vi "Laser_Setup_v1_v19 - Copy.vi"() -> ()   [LabVIEW 2019]
uses:
  <vilib>/Instr/_visa.llb/VISA Configure Serial Port (Instr).vi
panel:
  in  "Message":string
  in  "Arduino Functons":enum32{"DAC", "Step Motors", "TEC", "Settings"}(tab)=enum."Settings"
  in  "DAC: Show outputs value.":bool
  in  "DAC: Set VA.":bool
  in  "DAC: Set VB.":bool
  in  "DAC: Set VC.":bool
  in  "DAC: Set default outputs.":bool
  in  "DAC: Save outputs to DAC.":bool
  in  "DAC: Set VD.":bool
  in  "Step Motors: Reset Motor Y Position.":bool
  in  "Step Motors: Move Motor Y Forward.":bool
  in  "Step Motors: Move Motor X Forward.":bool
  in  "Step Motors: Reset Motor X Position.":bool
  in  "Step Motors: Move Motor Y Backward.":bool
  in  "Step Motors: Move Motor X Backward.":bool
  in  "Step Motors: Show Motor X Position.":bool
  in  "Step Motors: Show Motor Y Position.":bool
  in  "TEC: Get Firmware ID.":bool
  in  "TEC: Get Output Stage Status.":bool
  in  "TEC: Get Device Status.":bool
  in  "TEC: Set Output Stage Status ON.":bool
  in  "TEC: Set Output Stage Status OFF.":bool
  in  "TEC: Get if Temperature is Stable.":bool
  in  "TEC: Get Object Temperature Status.":bool
  in  "TEC: Do a Self Check.":bool
  in  "TEC: Get Error Status.":bool
  in  "TEC: Do Reset.":bool
  in  "TCP Settings":cluster{"Address":string, "Remote port":u16}={"Address"="192.168.4.1", "Remote port"=80}
  in  "Serial Settings":T1={"VISA resource name"="COM1", "baud rate"=9600, "data bits"=8, "parity"=enum."None", "stop bits"=10, "flow control"=0} {"flow control" items=["None"=0, "XON/XOFF"=1, "RTS/CTS"=2, "DTR/DSR"=4]; "stop bits" items=["1.0"=10, "1.5"=15, "2.0"=20]; "data bits" min=5 max=8 step=1; "baud rate" items=["75"=75, "110"=110, "134"=134, "150"=150, "300"=300, "600"=600, "1200"=1200, "1800"=1800, "2400"=2400, "4800"=4800, "7200"=7200, "9600"=9600, "14400"=14400, "19200"=19200, "28800"=28800, "38400"=38400, "56000"=56000, "57600"=57600, "115200"=115200, "128000"=128000, "230400"=230400]}
  in  "Start/Stop Communication":bool
  in  "Default Settings":bool
  in  "Stop VI":bool
  in  "Choose Communication":bool=TRUE
  in  "Main: Start Checks":bool
  out "Response":string
  # "Control Software of Laser Beam Test Bench \nversion 1.0"
  # "National and Kapodistrian University of Athens\nAerospace Inst Lab\n2021"
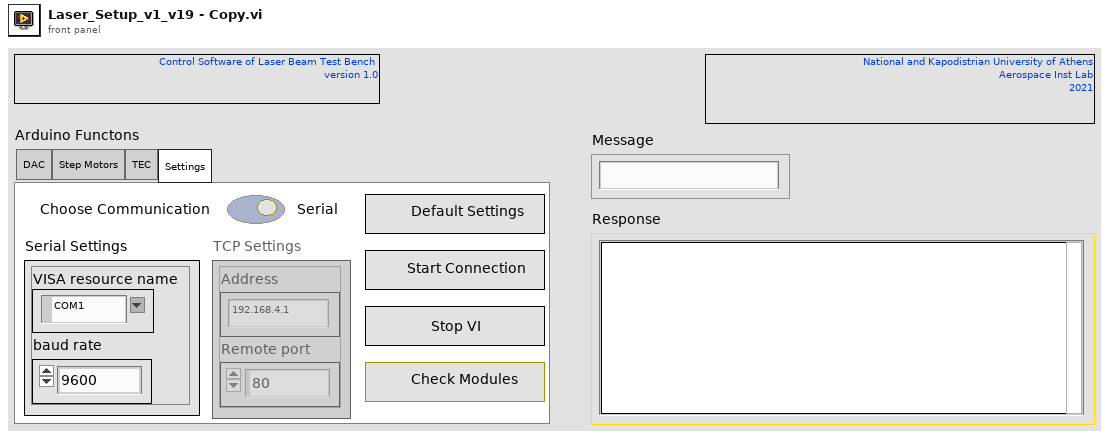
[diagram p1: front panel]
types:
  T1 = cluster{"VISA resource name":refnum<visa-resource-name>, "baud rate":u32, "data bits":u16, "parity":enum16{"None", "Odd", "Even", "Mark", "Space"}, "stop bits":u16, "flow control":u16}
  T2 = enum16{"Standard", "Buffered", "CRLF", "Immediate"}
  T3 = enum8{"Enabled", "Disabled", "Disabled and Grayed Out"}
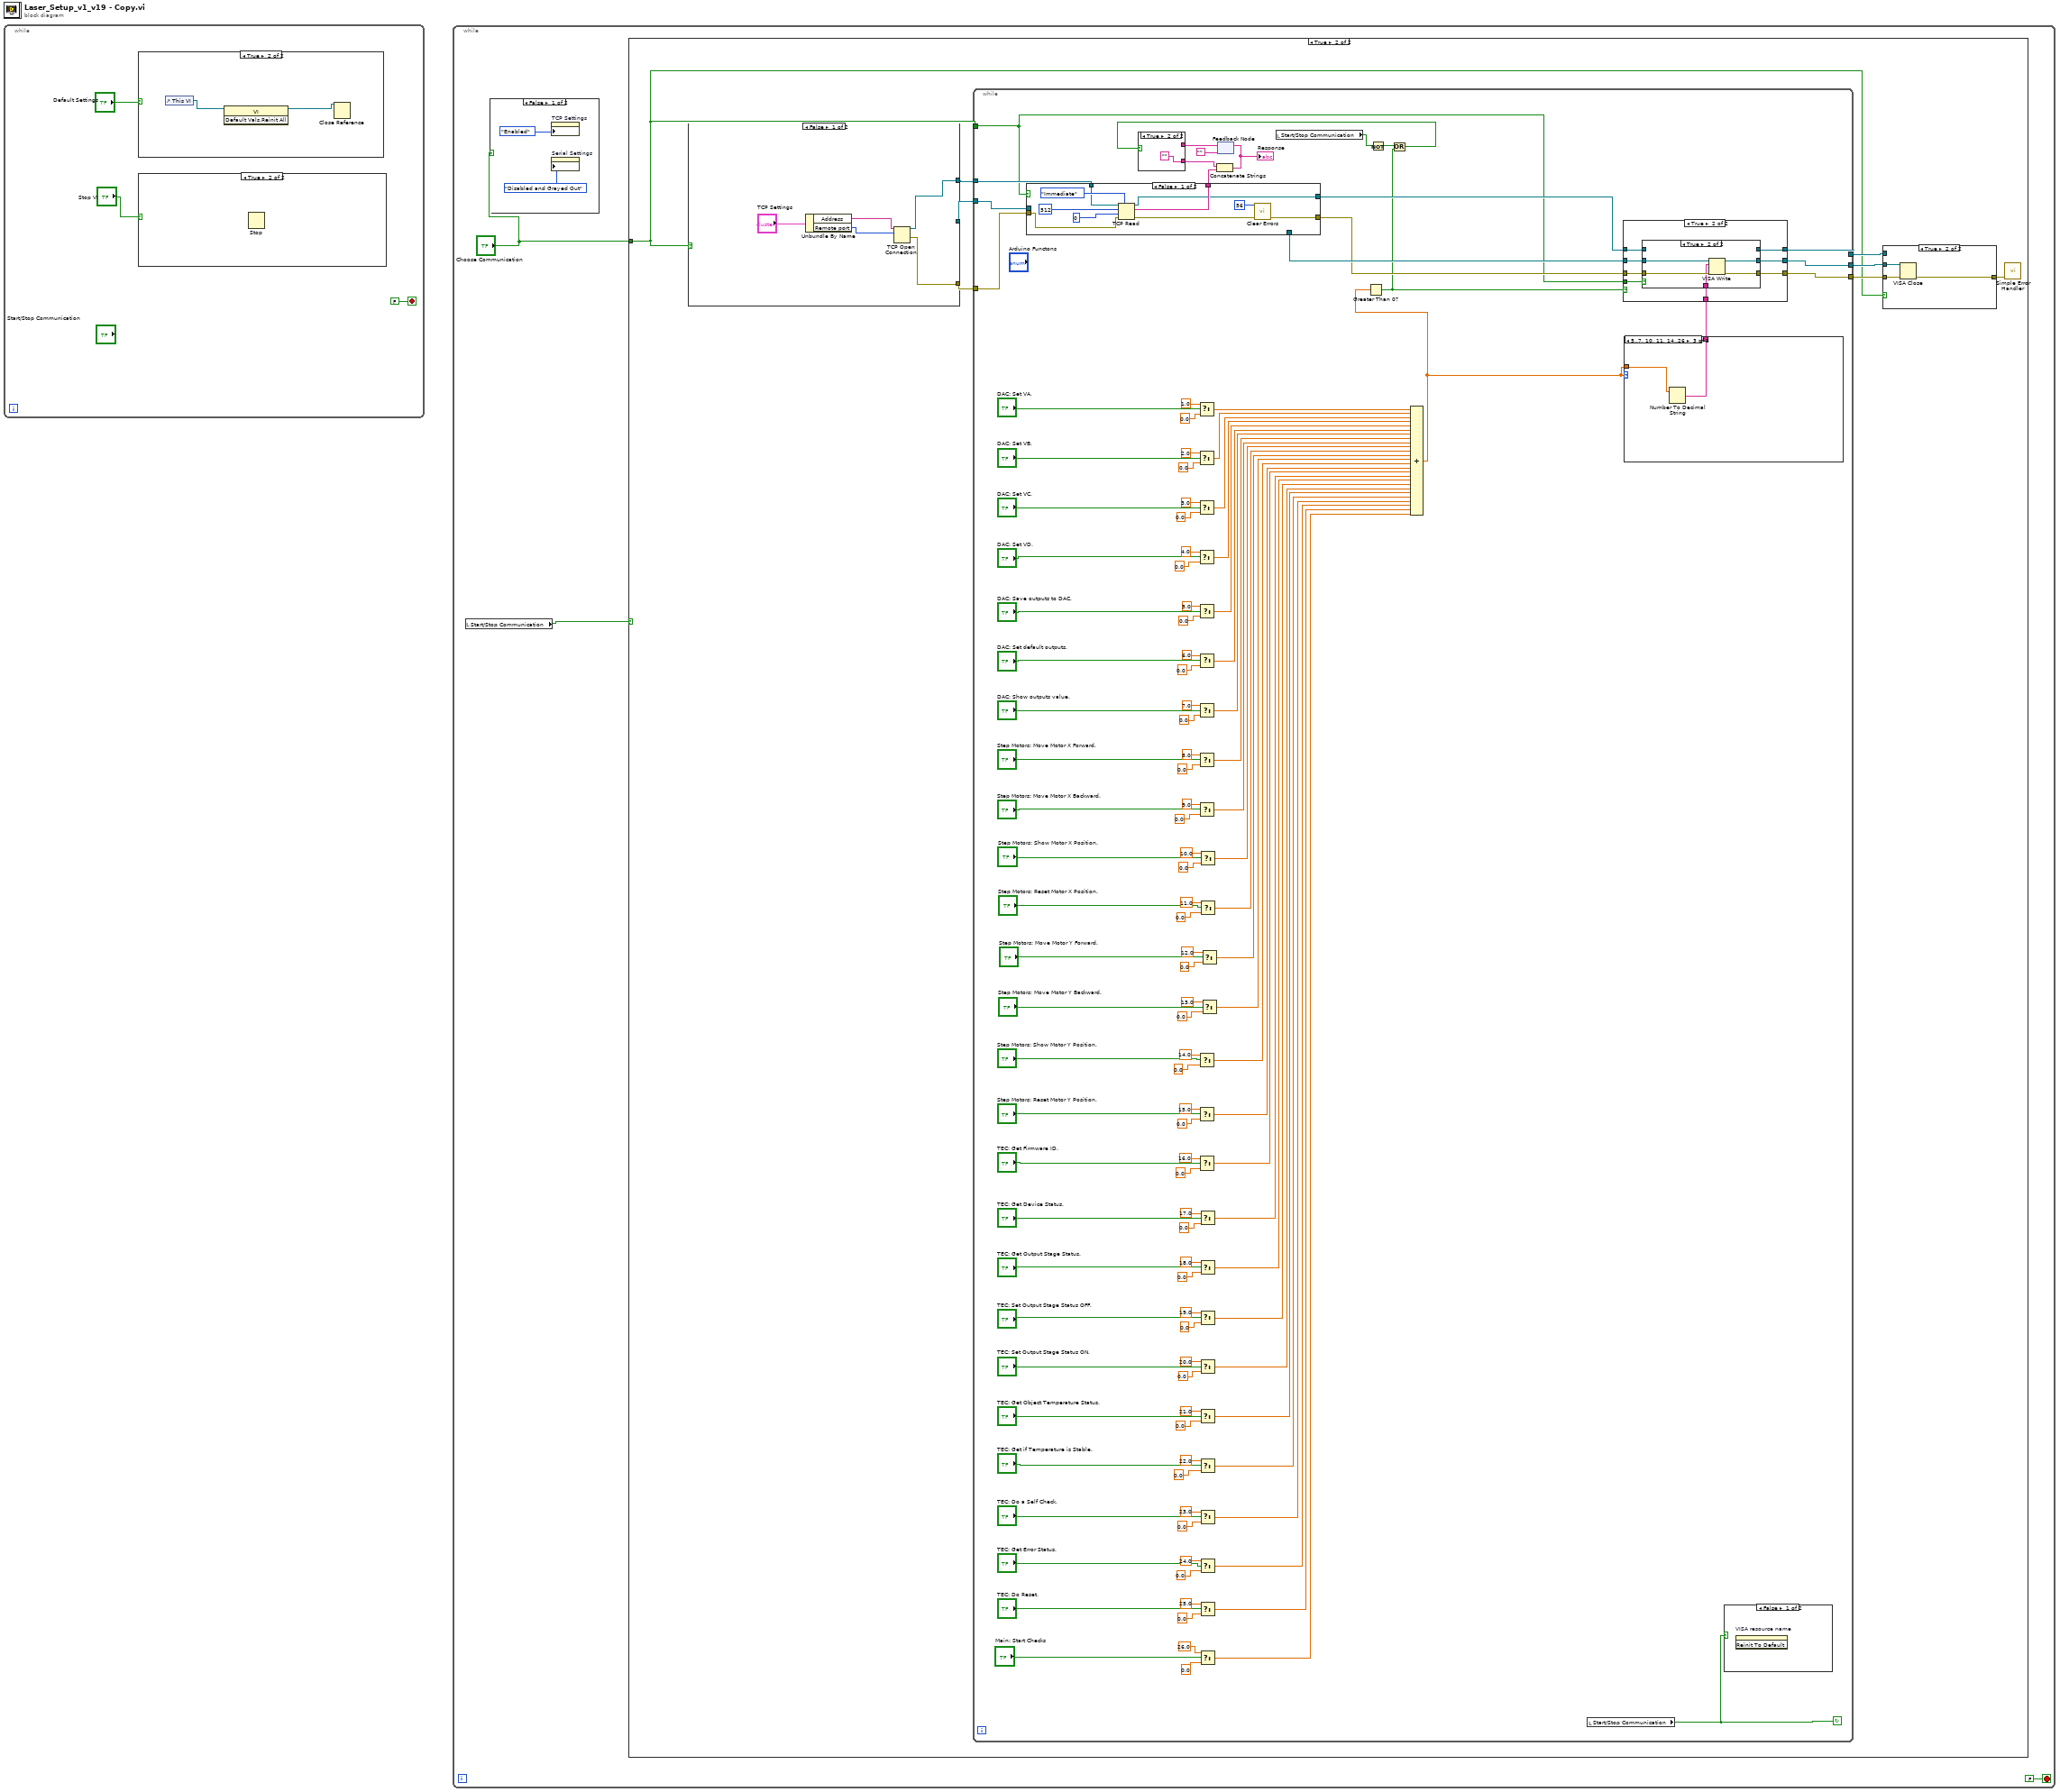
[diagram p0: block diagram]
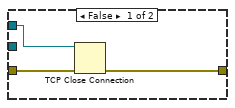
[diagram p5: hidden frame]
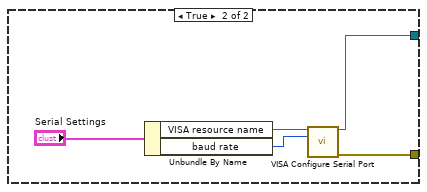
[diagram p6: hidden frame]
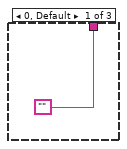
[diagram p7: hidden frame]
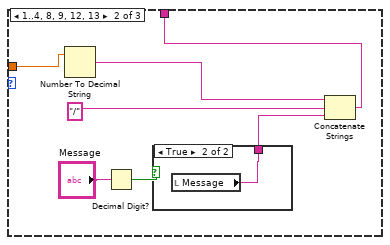
[diagram p8: hidden frame]
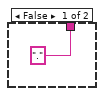
[diagram p9: hidden frame]
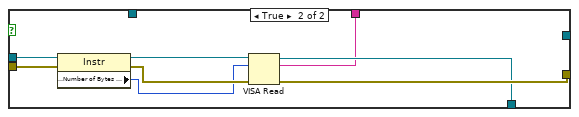
[diagram p11: hidden frame]
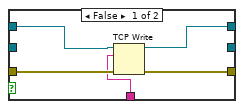
[diagram p14: hidden frame]
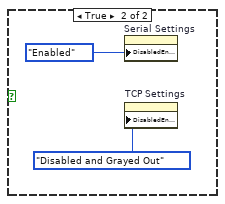
[diagram p15: hidden frame]
diagram:
  n1 = while {
    stop <- FALSE stop-if-true
    n2 = case shown="True" "Default Settings" {
      frame False {
      }
      frame True {
        n3 = control-ref of="This VI"() -> (w5:refnum<vi>)
        n4 = invoke class="VI" method="Default Vals.Reinit All"(reference=w5) -> (reference out=w4:refnum<vi>)  [unwired: 2 in, 2 out]
        n5 = Close Reference(reference=w4) -> ()  [unwired: 1 in, 1 out]
      }
    }
    n6 = case shown="True" "Stop VI" {
      frame False {
      }
      frame True {
        n7 = Stop() -> ()  [unwired: 1 in]
      }
    }
  }
  n8 = while {
    stop <- FALSE stop-if-true
    n9 = local read "Start/Stop Communication"() -> (w7:bool)
    n10 = case shown="False" "Choose Communication" {
      frame False {
        n11 = property on="TCP Settings" class="Clust (strict)"("DisabledEnum"=T3."Enabled" ("Disabled")) -> ()  [unwired: 2 in, 2 out]
        n12 = property on="Serial Settings" class="Clust (strict)"("DisabledEnum"=T3."Disabled and Grayed Out" ("Disabled")) -> ()  [unwired: 2 in, 2 out]
      }
      frame True {
        n13 = property on="Serial Settings" class="Clust (strict)"("DisabledEnum"=T3."Enabled" ("Disabled")) -> ()  [unwired: 2 in, 2 out]
        n14 = property on="TCP Settings" class="Clust (strict)"("DisabledEnum"=T3."Disabled and Grayed Out" ("Disabled")) -> ()  [unwired: 2 in, 2 out]
      }
    }
    n15 = case shown="True" w7 {
      tunnel: "Choose Communication" -> [_ w9]
      frame False {
      }
      frame True {
        n16 = case shown="False" w9 {
          tunnel: [_ w31] -> w16
          tunnel: [w27 w30] -> w15
          tunnel: [w23 _] -> w11
          frame False {
            n17 = Unbundle By Name("TCP Settings") -> ("Address"=w25:string, "Remote port"=w24:u16)
            n18 = TCP Open Connection(address=w25, remote port or service name=w24) -> (connection ID=w23:refnum<k5>, error out=w27:errorcluster)  [unwired: 3 in]
          }
          frame True {
            n19 = Unbundle By Name("Serial Settings") -> ("VISA resource name"=w29:refnum<visa-resource-name>, "baud rate"=w32:u32)
            n20 = call-poly "VISA Configure Serial Port"("VISA resource name"=w29, "baud rate (9600)"=w32) -> ("VISA resource name out"=w31:refnum<visa-resource-name>, "error out"=w30:errorcluster)  [unwired: 7 in, 5 out]
          }
        }
        n21 = while {
          tunnel: w16 -> [w156]
          tunnel: w15 -> [w155]
          tunnel: [w158] -> w13
          tunnel: [w157] -> w12
          tunnel: w11 -> [w147]
          tunnel: [w145] -> w10
          tunnel: w9 -> [w144]
          stop <- w143 continue-if-true
          n22 = case shown="False" w144 {
            tunnel: [w173 w186] -> w148
            tunnel: w156 -> [_ w185]
            tunnel: w155 -> [w174 w184]
            tunnel: [_ w183] -> w154
            tunnel: [w177 w181] -> w152
            tunnel: w147 -> [w172 _]
            tunnel: [w171 _] -> w146
            frame False {
              n23 = TCP Read(connection ID=w172, bytes to read=512, error in (no error)=w174, 7:T2."Immediate" ("mode (standard)"), 9:0 ("timeout ms (25000)")) -> (connection ID out=w171:refnum<k5>, data out=w177:string, error out=w175:errorcluster)
              n24 = call <vilib>:"Clear Errors.vi"("error in (no error)"=w175, "specific error code to clear (0: all)"=56) -> ("error out"=w173:errorcluster)  [unwired: 4 in, 1 out]
            }
            frame True {
              n25 = property class="Instr"(reference=w185, error in=w184) -> (reference out=w188:refnum<visa-resource-name>, error out=w187:errorcluster, "Serial Settings:Number of Bytes at Serial Port"=w182:u32)
              n26 = VISA Read(VISA resource name=w188, byte count=w182, error in (no error)=w187) -> (VISA resource name out=w183:refnum<visa-resource-name>, read buffer=w181:string, error out=w186:errorcluster)  [unwired: 1 out]
            }
          }
          n27 = Select(t=1.0, s="DAC: Set VA.", f=0.0) -> (s? t:f=w91:dbl)
          n28 = Select(t=2.0, s="DAC: Set VB.", f=0.0) -> (s? t:f=w97:dbl)
          n29 = Select(t=3.0, s="DAC: Set VC.", f=0.0) -> (s? t:f=w96:dbl)
          n30 = Select(t=4.0, s="DAC: Set VD.", f=0.0) -> (s? t:f=w95:dbl)
          n31 = Select(t=5.0, s="DAC: Save outputs to DAC.", f=0.0) -> (s? t:f=w94:dbl)
          n32 = Select(t=6.0, s="DAC: Set default outputs.", f=0.0) -> (s? t:f=w93:dbl)
          n33 = Select(t=7.0, s="DAC: Show outputs value.", f=0.0) -> (s? t:f=w92:dbl)
          n34 = Select(t=8.0, s="Step Motors: Move Motor X Forward.", f=0.0) -> (s? t:f=w79:dbl)
          n35 = Select(t=9.0, s="Step Motors: Move Motor X Backward.", f=0.0) -> (s? t:f=w78:dbl)
          n36 = Select(t=14.0, s="Step Motors: Show Motor Y Position.", f=0.0) -> (s? t:f=w73:dbl)
          n37 = Select(t=15.0, s="Step Motors: Reset Motor Y Position.", f=0.0) -> (s? t:f=w72:dbl)
          n38 = Select(t=16.0, s="TEC: Get Firmware ID.", f=0.0) -> (s? t:f=w71:dbl)
          n39 = Select(t=17.0, s="TEC: Get Device Status.", f=0.0) -> (s? t:f=w70:dbl)
          n40 = Select(t=18.0, s="TEC: Get Output Stage Status.", f=0.0) -> (s? t:f=w69:dbl)
          n41 = Select(t=19.0, s="TEC: Set Output Stage Status OFF.", f=0.0) -> (s? t:f=w68:dbl)
          n42 = Select(t=20.0, s="TEC: Set Output Stage Status ON.", f=0.0) -> (s? t:f=w67:dbl)
          n43 = Select(t=21.0, s="TEC: Get Object Temperature Status.", f=0.0) -> (s? t:f=w66:dbl)
          n44 = Select(t=22.0, s="TEC: Get if Temperature is Stable.", f=0.0) -> (s? t:f=w65:dbl)
          n45 = Select(t=23.0, s="TEC: Do a Self Check.", f=0.0) -> (s? t:f=w64:dbl)
          n46 = Select(t=24.0, s="TEC: Get Error Status.", f=0.0) -> (s? t:f=w63:dbl)
          n47 = Select(t=25.0, s="TEC: Do Reset.", f=0.0) -> (s? t:f=w62:dbl)
          n48 = Select(t=26.0, s="Main: Start Checks", f=0.0) -> (s? t:f=w61:dbl)
          n49 = Select(t=10.0, s="Step Motors: Show Motor X Position.", f=0.0) -> (s? t:f=w77:dbl)
          n50 = Select(t=11.0, s="Step Motors: Reset Motor X Position.", f=0.0) -> (s? t:f=w76:dbl)
          n51 = Select(t=12.0, s="Step Motors: Move Motor Y Forward.", f=0.0) -> (s? t:f=w75:dbl)
          n52 = Select(t=13.0, s="Step Motors: Move Motor Y Backward.", f=0.0) -> (s? t:f=w74:dbl)
          n53 = feedback #1("") -> (w150:string)
          n54 = local read "Start/Stop Communication"() -> (w142:bool)
          n55 = Not(x=w142) -> (.not. x?=w141:bool)
          n56 = Compound Arithmetic op=ADD(w91, w97, w96, w95, w94, w93, w92, w79, w78, w77, w76, w75, w74, w73, w72, w71, w70, w69, w68, w67, w66, w65, w64, w63, w62, w61) -> (w60:dbl)
          n57 = Greater Than 0?(x=w60) -> (x > 0?=w139:bool)
          n58 = Or(x=w141, y=w139) -> (x .or. y?=w140:bool)
          n59 = case shown="True" w140 {
            tunnel: w150 -> [w189 _]
            tunnel: [w189 ""] -> w149
            frame False {
            }
            frame True {
            }
          }
          n60 = Concatenate Strings(w149, w152) -> (w151:string)
          "Response" <- w151
          n61 = feedback-in #1(w151) -> ()
          n62 = local read "Start/Stop Communication"() -> (w143:bool)
          n63 = case shown="5..7, 10, 11, 14..26" w60 {
            tunnel: ["" w163 w170] -> w98
            tunnel: w60 -> [_ w164 w169]
            frame 0, Default {
            }
            frame 1..4, 8, 9, 12, 13 {
              n64 = Number To Decimal String(number=w164) -> (decimal integer string=w166:string)  [unwired: 1 in]
              n65 = Decimal Digit?(1:"Message") -> (0:w161:bool)
              n66 = case shown="True" w161 {
                tunnel: ["." w168] -> w162
                frame False {
                }
                frame True {
                  n67 = local read "Message"() -> (w168:string)
                }
              }
              n68 = Concatenate Strings(w166, "/", w162) -> (w163:string)
            }
            frame 5..7, 10, 11, 14..26 {
              n69 = Number To Decimal String(number=w169) -> (decimal integer string=w170:string)  [unwired: 1 in]
            }
          }
          n70 = case shown="True" w139 {
            tunnel: w148 -> [w193 w201]
            tunnel: [w193 w200] -> w158
            tunnel: w154 -> [w192 w199]
            tunnel: [w192 w198] -> w157
            tunnel: w146 -> [w191 w197]
            tunnel: [w191 w196] -> w145
            tunnel: w144 -> [_ w195]
            tunnel: w98 -> [_ w194]
            frame False {
            }
            frame True {
              n71 = case shown="True" w195 {
                tunnel: w201 -> [w206 w211]
                tunnel: [w205 w210] -> w200
                tunnel: w199 -> [_ w209]
                tunnel: [_ w208] -> w198
                tunnel: w197 -> [w204 _]
                tunnel: [w203 _] -> w196
                tunnel: w194 -> [w202 w207]
                frame False {
                  n72 = TCP Write(connection ID=w204, data in=w202, error in (no error)=w206) -> (connection ID out=w203:refnum<k5>, error out=w205:errorcluster)  [unwired: 1 in, 1 out]
                }
                frame True {
                  n73 = VISA Write(VISA resource name=w209, write buffer=w207, error in (no error)=w211) -> (VISA resource name out=w208:refnum<visa-resource-name>, error out=w210:errorcluster)  [unwired: 1 out]
                }
              }
            }
          }
          n74 = case shown="False" w143 {
            frame False {
              n75 = invoke on="VISA resource name" class="VISAName" method="Reinit To Default"() -> ()  [unwired: 3 in, 3 out]
            }
            frame True {
            }
          }
        }
        n76 = case shown="True" w9 {
          tunnel: [w18 w22] -> w14
          tunnel: w13 -> [w19 w21]
          tunnel: w12 -> [_ w20]
          tunnel: w10 -> [w17 _]
          frame False {
            n77 = TCP Close Connection(connection ID=w17, error in (no error)=w19) -> (error out=w18:errorcluster)  [unwired: 2 out]
          }
          frame True {
            n78 = VISA Close(VISA resource name=w20, error in (no error)=w21) -> (error out=w22:errorcluster)
          }
        }
        n79 = call <vilib>:"Simple Error Handler.vi"("error in (no error)"=w14) -> ()  [unwired: 1 in, 8 out]
      }
    }
  }
